vi "Check For Messages.vi"(11 "data in":u8[](array[numeric])) -> (2 "PDU valid?":bool, 3 "data":u8[](array[numeric]))   [LabVIEW 2021, in "ELAN Data Unit.lvclass"]
uses:
  ELAN Data Unit.lvclass
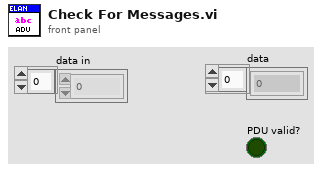
[diagram p1: front panel]
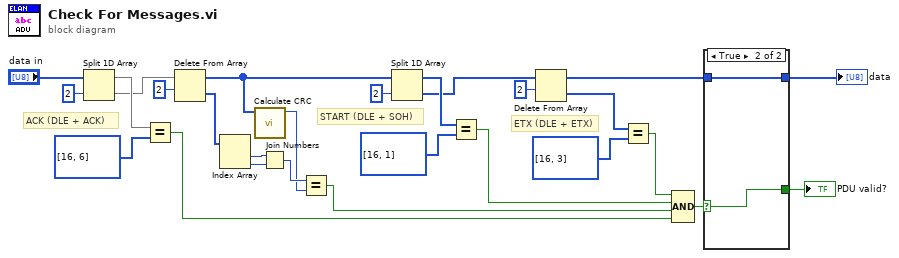
[diagram p0: block diagram]
diagram:
  # "START (DLE + SOH)"
  # "ETX (DLE + ETX)"
  # "ACK (DLE + ACK)"
  n1 = Split 1D Array(array="data in", index=2) -> (first subarray=w24:u8[], second subarray=w5:u8[])
  n2 = Equal?(x=w24, y=u8[] [16, 6] ("data")) -> (x = y?=w9:bool)
  n3 = Delete From Array(array=w5, length=2) -> (deleted portion=w22:u8[], array with subset deleted=w1:u8[])  [unwired: 1 in]
  n4 = Index Array(array=w22) -> (element #1=w15:u8, element #2=w14:u8)  [unwired: 2 in]
  n5 = call "Calculate CRC.vi"("data"=w1) -> ("CRC-16"=w7:u16)  [unwired: 10 in]
  n6 = Join Numbers(hi=w15, lo=w14) -> ((hi.lo)=w8:u16)
  n7 = Equal?(x=w8, y=w7) -> (x = y?=w2:bool)
  n8 = Split 1D Array(array=w1, index=2) -> (first subarray=w12:u8[], second subarray=w4:u8[])
  n9 = Equal?(x=w12, y=u8[] [16, 1] ("data")) -> (x = y?=w3:bool)
  n10 = Delete From Array(array=w4, length=2) -> (deleted portion=w19:u8[], array with subset deleted=w6:u8[])  [unwired: 1 in]
  n11 = Equal?(x=w19, y=u8[] [16, 3] ("data")) -> (x = y?=w10:bool)
  n12 = Compound Arithmetic op=AND(w10, w3, w2, w9) -> (w17:bool)
  n13 = case shown="True" w17 {
    selector: w17 -> [_ w28]
    tunnel: w6 -> [_ w29]
    tunnel: [_ w29] -> w18
    tunnel: [_ w28] -> w16
    frame False {
    }
    frame True {
    }
  }
  "data" <- w18
  "PDU valid?" <- w16
